vi "Stop Core.vi"(10 "final error code":i32, 11 "Calculator Actor in":refnum<class "Calculator Actor.lvclass">) -> (3 "Calculator Actor out":refnum<class "Calculator Actor.lvclass">)   [LabVIEW 2015, in "Calculator Actor.lvclass"]
doc: "(<B>Filename</B>: Actor Framework.lvlib:Actor.lvclass:Stop Core.vi)\n\nDefines what the actor does before it stops. Use the <B>final error code</B> input to determine whether the actor shut down in response to an error.\n\nBy default, this method does nothing. A descendant class may override it to define behavior, such as shutting down any processes the actor initiated in its override of the Actor Core method."
uses:
  Calculator Actor.lvclass
  Calculator Actor.lvclass/Calculator Actor.ctl
  <vilib>/ActorFramework/Actor/Actor.lvclass
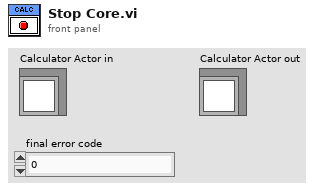
[diagram p1: front panel]
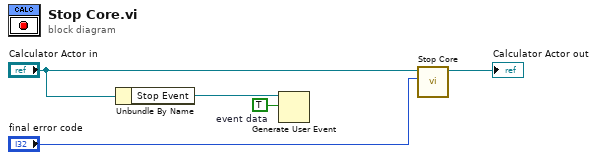
[diagram p0: block diagram]
diagram:
  w1 = TRUE  # event data
  n1 = Unbundle By Name("Calculator Actor in") -> ("Stop Event"=w2:refnum<user-event>)
  n2 = Generate User Event(user event=w2, event data cluster=w1) -> ()  [unwired: 2 in, 2 out]
  n3 = call-parent "Stop Core.vi"("final error code"="final error code", "Actor in"="Calculator Actor in") -> ("Actor out"=→"Calculator Actor out":refnum<class "Calculator Actor.lvclass">)  [unwired: 9 in]
